vi "Close CITI File.vi"(8 "error in (no error)":errorcluster, 11 "CITI reference in":refnum<k24>) -> (0 "error out":errorcluster)   [LabVIEW 2023, in "NI_HFNetworkAnalysis.lvlib"]
doc: "Close reference to the CITI file.\n\n<b>Note</b>\nUse <b>Save CITI File.vi</b> to save the CITI packages in memory to file before closing the CITI file reference."
uses:
  NI_HFNetworkAnalysis.lvlib
  C:/srd-semi-rfcal-software/AuxTools/STSRFFixtureCharactUtility/Source/Code Modules/Fixture/Dependencies/HFNetworkAnalysis/Support Files/NACE.Utils.Data.dll
  Support Files/NACE.Utils.Data.dll
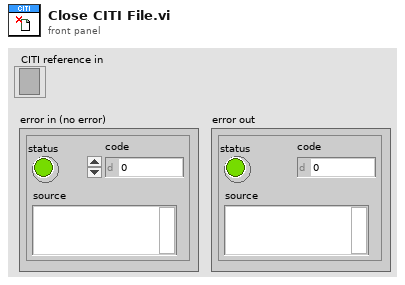
[diagram p1: front panel]
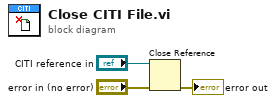
[diagram p0: block diagram]
diagram:
  n1 = Close Reference(reference="CITI reference in", error in (no error)="error in (no error)") -> (error out=→"error out":errorcluster)
